vi "RTP_RTSP - TEARDOWN - METHOD.vi"(0 "RTSP Session":T1, 9 "timeout ms (1000)":i32=1000, 11 "error in (no error)":errorcluster) -> (4 "RTSP Session 2":T1, 15 "error out":errorcluster)   [LabVIEW 2014]
uses:
  RTSP Session.ctl
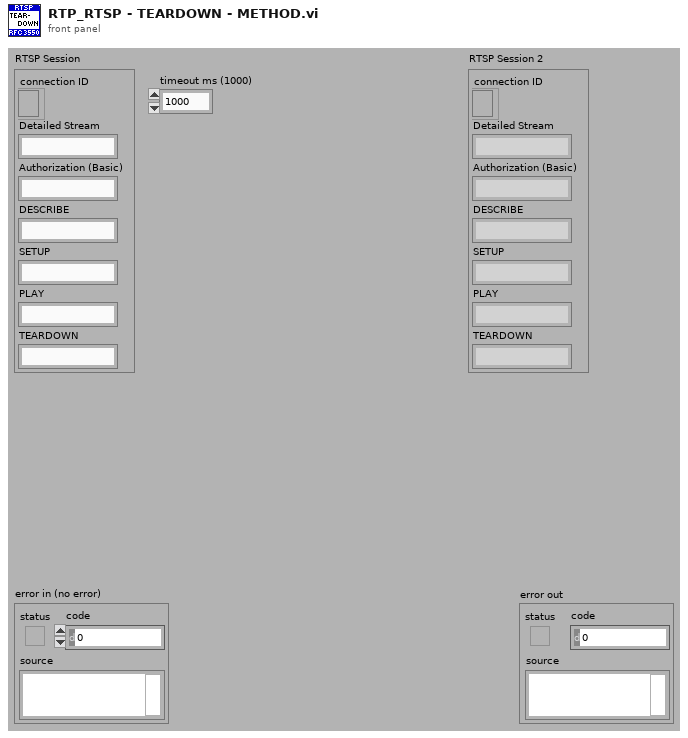
[diagram p1: front panel]
types:
  T1 = typedef "RTSP Session.ctl" = cluster{"connection ID":refnum<k5>, "Authorization (Basic)":string, "Detailed Stream":string, "DESCRIBE":string, "SETUP":string, "PLAY":string, "TEARDOWN":string}
  T2 = enum16{"Standard", "Buffered", "CRLF", "Immediate"}
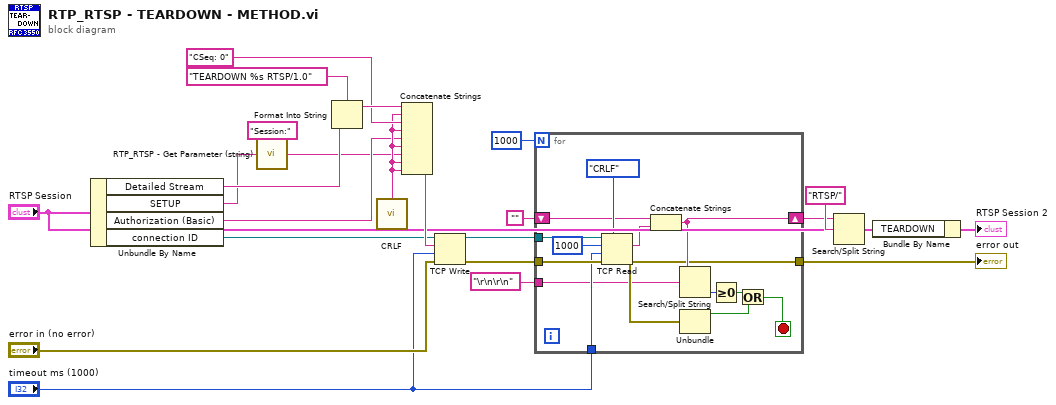
[diagram p0: block diagram]
diagram:
  n1 = Unbundle By Name("RTSP Session") -> ("Detailed Stream"=w9:string, "SETUP"=w6:string, "Authorization (Basic)"=w8:string, "connection ID"=w10:refnum<k5>)
  n2 = call "RTP_RTSP - Get Parameter (string).vi"("Name"="Session:" ("search string/char (-)"), "Data"=w6) -> ("Parameter"=w1:string)  [unwired: 13 in]
  n3 = Format Into String(format string="TEARDOWN %s RTSP/1.0", w9) -> (resulting string=w22:string)  [unwired: 2 in, 1 out]
  n4 = call "CRLF.vi"() -> ("CRLF"=w11:string)
  n5 = Concatenate Strings(w22, w11, "CSeq: 0" ("string"), w11, w8, w11, w1, w11, w11) -> (w21:string)
  n6 = TCP Write(connection ID=w10, data in=w21, error in (no error)="error in (no error)", 9:"timeout ms (1000)") -> (connection ID out=w17:refnum<k5>, error out=w16:errorcluster)  [unwired: 1 out]
  n7 = for {
    N: 1000 -> [_]
    tunnel: w16 -> [w38]
    tunnel: w17 -> [w37]
    tunnel: [w29] -> w14
    shift-right: [w31] -> w12
    shift-left: "" -> [w35]
    tunnel: "timeout ms (1000)" -> [w32]
    tunnel: "\r\n\r\n" ("search string/char (-)") -> [w28]
    stop <- w25 stop-if-true
    n8 = TCP Read(connection ID=w37, bytes to read=1000, error in (no error)=w38, 7:T2."CRLF" ("mode (standard)"), 9:w32) -> (data out=w34:string, error out=w29:errorcluster)  [unwired: 1 out]
    n9 = Concatenate Strings(w35, w34) -> (w31:string)
    n10 = Search/Split String(string=w31, search string/char (-)=w28) -> (offset of match=w30:i32)  [unwired: 1 in, 2 out]
    n11 = Unbundle(w29) -> ("status"=w26:bool)  [unwired: 2 out]
    n12 = Greater Or Equal To 0?(x=w30) -> (x >= 0?=w27:bool)
    n13 = Or(x=w27, y=w26) -> (x .or. y?=w25:bool)
  }
  "error out" <- w14
  n14 = Search/Split String(string=w12, search string/char (-)="RTSP/") -> (match + rest of string=w2:string)  [unwired: 1 in, 2 out]
  n15 = Bundle By Name(cluster="RTSP Session", "TEARDOWN"=w2) -> (→"RTSP Session 2":T1)
